vi "Wait for Invocation.vi"(8 "error in (no error)":errorcluster, 10 "timeout in ms (-1)":i32, 11 "WAMP Client in":refnum<class "WAMP Client.lvclass">) -> (0 "error out":errorcluster, 1 "timed out?":bool, 2 "WAMP Invocation":T1, 3 "WAMP Client out":refnum<class "WAMP Client.lvclass">)   [LabVIEW 2021, in "wamplv.lvlib" / "WAMP Client.lvclass"]
doc: "Waits for a WAMP invocation call"
uses:
  WAMP Client.lvclass
  TypeDefs/INVOCATION payload.ctl
  Invocation Request ID/Invocation Request ID.lvclass
  WAMP Client.lvclass/WAMP Client.ctl
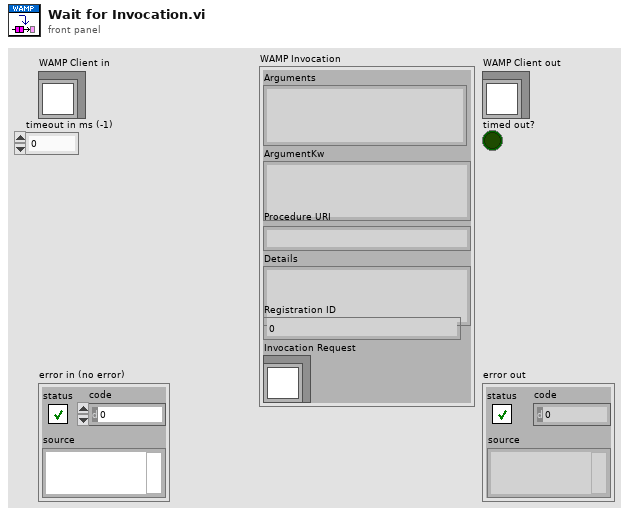
[diagram p1: front panel]
types:
  T1 = typedef "wamplv.lvlib/WAMP Client.lvclass/INVOCATION payload.ctl" = cluster{"Arguments":string, "ArgumentKw":string, "Procedure URI":string, "Details":string, "Registration ID":u64, "Invocation Request":refnum<class "Invocation Request ID.lvclass">}
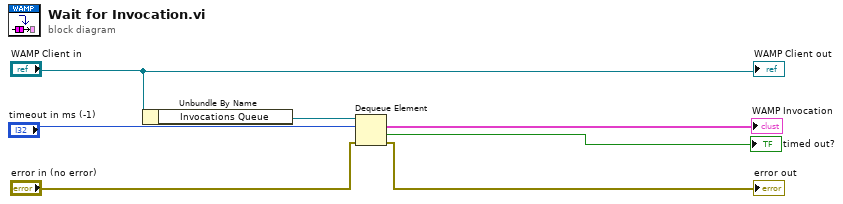
[diagram p0: block diagram]
diagram:
  n1 = Unbundle By Name("WAMP Client in") -> ("Invocations Queue"=w6:refnum<queue>)
  n2 = Dequeue Element(queue=w6, timeout in ms (-1)="timeout in ms (-1)", error in (no error)="error in (no error)") -> (element=→"WAMP Invocation":T1, timed out?=→"timed out?":bool, error out=→"error out":errorcluster)  [unwired: 1 out]
  "WAMP Client out" <- "WAMP Client in"
